vi "FPGA Main.vi"() -> ()   [LabVIEW 2022 SP3]
uses:
  <vilib>/rvi/Emulation/niFpgaGetClockAttributes.vi
  <vilib>/rvi/Emulation/niFpgaSctlEmulationGetInTimedLoop.vi
  <vilib>/rvi/Emulation/niFpgaEmulationReportErrorSimple.vi
  <vilib>/rvi/eio/common/nirviEmuTemplateMethod_errors.vi
  <vilib>/rvi/Emulation/niFpgaCriticalErrorInLSC.vi
  <vilib>/eio/EIONode/EIONode.xnode
panel:
  out "Counter Register":u64
  out "布尔":bool
  out "Counters":u64
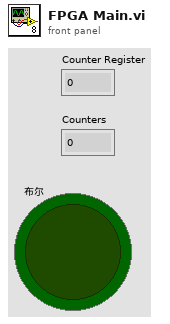
[diagram p1: front panel]
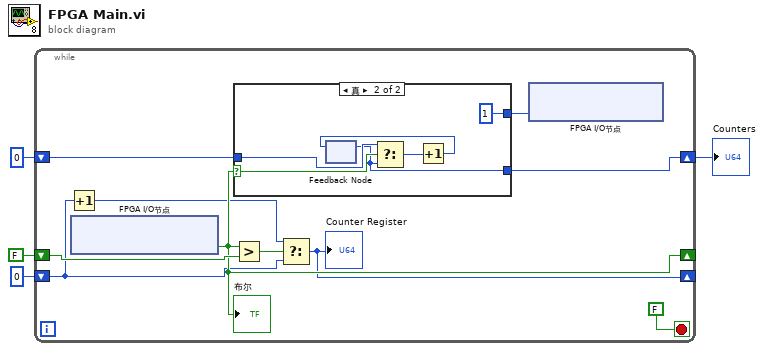
[diagram p0: block diagram]
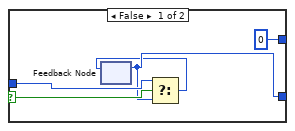
[diagram p2: hidden frame]
diagram:
  n1 = while {
    shift-right: [w11] -> w3
    shift-left: i16 0 -> [w12]
    shift-right: [w9] -> _
    shift-left: FALSE -> [w10]
    shift-right: [w5] -> _
    shift-left: u64 0 -> [w6]
    stop <- FALSE stop-if-true
    n2 = Increment(x=w6) -> (x+1=w7:u64)
    n3 = xnode "FPGA I/O节点"() -> ("USER Push Button"=w9:bool)  [unwired: 1 in, 1 out]
    "布尔" <- w9
    n4 = case shown="真" w9 {
      selector: w9 -> [w18 w22]
      tunnel: [i16 0 i16 1] -> w13
      tunnel: w12 -> [w17 w21]
      tunnel: [w16 w20] -> w11
      frame False {
        n5 = feedback #1() -> (w16:i16)  [unwired: 1 in]
        n6 = Select(t=w17, s=w18, f=w16) -> (s? t:f=w15:i16)
        n7 = feedback-in #1(w15) -> ()
      }
      frame True {
        n8 = feedback #2() -> (w20:i16)  [unwired: 1 in]
        n9 = Select(t=w21, s=w22, f=w20) -> (s? t:f=w24:i16)
        n10 = Increment(x=w24) -> (x+1=w23:i16)
        n11 = feedback-in #2(w23) -> ()
      }
    }
    n12 = Greater?(x=w9, y=w10) -> (0:w8:bool)
    n13 = Select(t=w7, s=w8, f=w6) -> (s? t:f=w5:u64)
    "Counter Register" <- w5
    n14 = xnode "FPGA I/O节点"("USER FPGA LED"=w13) -> ()  [unwired: 1 in, 1 out]
  }
  "Counters" <- w3
